vi "test_Get Channel Connection (2010).vi"(8 "error in (no error)":errorcluster) -> (0 "error out":errorcluster)   [LabVIEW 2020, in "Test_Routing Templates.lvlib"]
uses:
  Test_Routing Templates.lvlib
  Connection Lookups/2010 Connection Lookup/2010 Connection Lookup.lvclass
  <vilib>/addons/_JKI Toolkits/Caraya/classes/Assert/Assert Equal Value_Variant.vi
  <vilib>/addons/_JKI Toolkits/Caraya/classes/Assert/Assert Error.vi
  <vilib>/addons/_JKI Toolkits/Caraya/classes/Test/Test.lvclass
  <vilib>/addons/_JKI Toolkits/Caraya/classes/Assert/Assert.lvclass
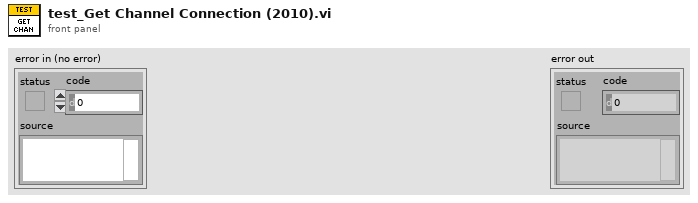
[diagram p1: front panel]
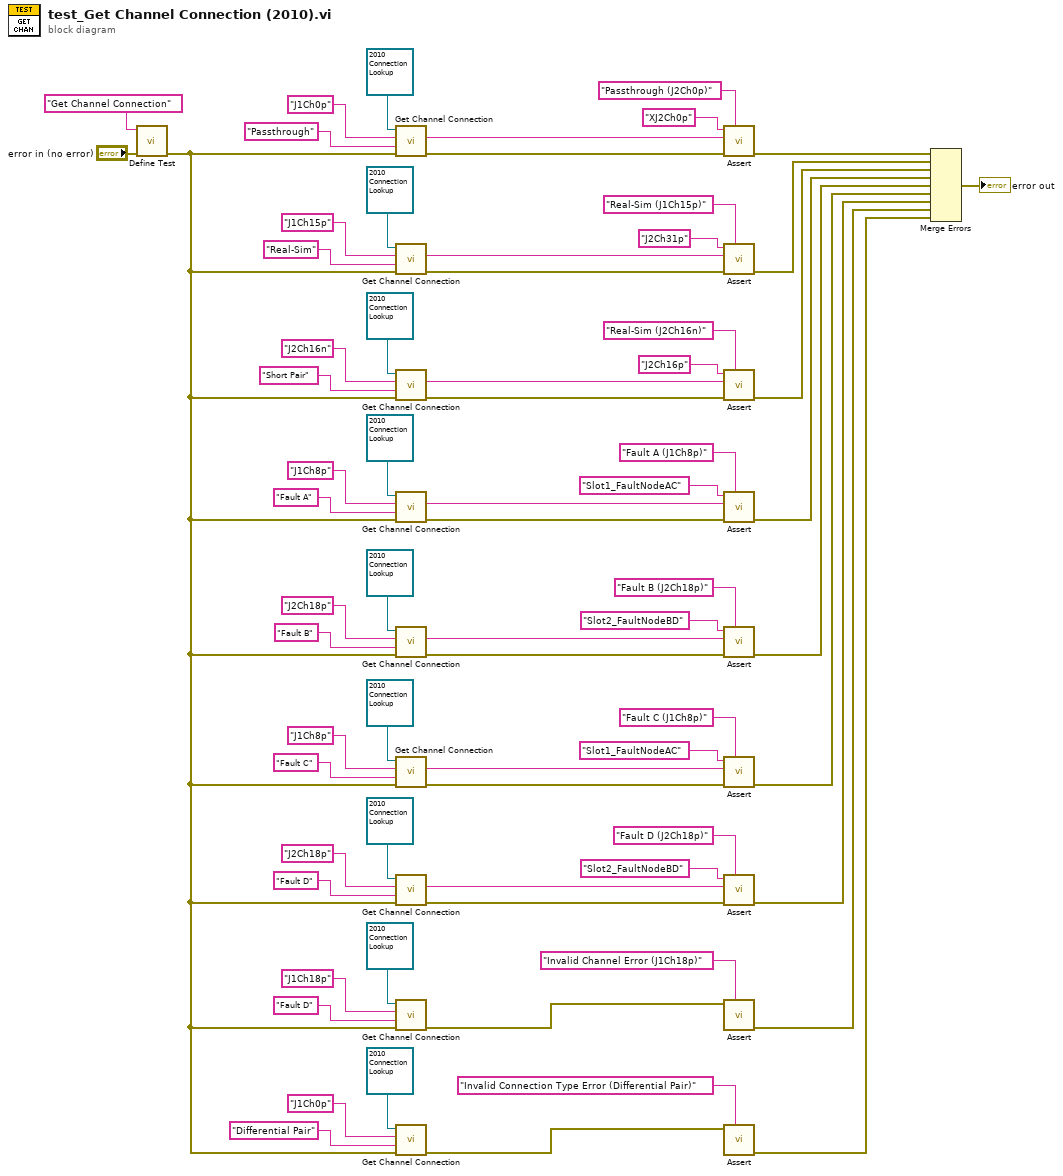
[diagram p0: block diagram]
diagram:
  n1 = call <vilib>:"Define Test.vi"("error in (no error)"="error in (no error)", "Label (VI Title)"="Get Channel Connection") -> ("error out"=w9:errorcluster)  [unwired: 9 in]
  n2 = call-dynamic "Get Channel Connection.vi"("error in (no error)"=w9, "Connection Type"="Passthrough", "Channel"="J1Ch0p", "2010 Connection Lookup in"=refnum<class "2010 Connection Lookup.lvclass"> refnum) -> ("error out"=w70:errorcluster, "Connected Channel"=w63:string)  [unwired: 5 in, 1 out]
  n3 = call-dynamic "Get Channel Connection.vi"("error in (no error)"=w9, "Connection Type"="Real-Sim", "Channel"="J1Ch15p", "2010 Connection Lookup in"=refnum<class "2010 Connection Lookup.lvclass"> refnum) -> ("error out"=w56:errorcluster, "Connected Channel"=w60:string)  [unwired: 5 in, 1 out]
  n4 = call-dynamic "Get Channel Connection.vi"("error in (no error)"=w9, "Connection Type"="Short Pair", "Channel"="J2Ch16n", "2010 Connection Lookup in"=refnum<class "2010 Connection Lookup.lvclass"> refnum) -> ("error out"=w53:errorcluster, "Connected Channel"=w49:string)  [unwired: 5 in, 1 out]
  n5 = call-dynamic "Get Channel Connection.vi"("error in (no error)"=w9, "Connection Type"="Fault A", "Channel"="J1Ch8p", "2010 Connection Lookup in"=refnum<class "2010 Connection Lookup.lvclass"> refnum) -> ("error out"=w42:errorcluster, "Connected Channel"=w46:string)  [unwired: 5 in, 1 out]
  n6 = call-dynamic "Get Channel Connection.vi"("error in (no error)"=w9, "Connection Type"="Fault B", "Channel"="J2Ch18p", "2010 Connection Lookup in"=refnum<class "2010 Connection Lookup.lvclass"> refnum) -> ("error out"=w39:errorcluster, "Connected Channel"=w35:string)  [unwired: 5 in, 1 out]
  n7 = call-dynamic "Get Channel Connection.vi"("error in (no error)"=w9, "Connection Type"="Fault C", "Channel"="J1Ch8p", "2010 Connection Lookup in"=refnum<class "2010 Connection Lookup.lvclass"> refnum) -> ("error out"=w32:errorcluster, "Connected Channel"=w28:string)  [unwired: 5 in, 1 out]
  n8 = call-dynamic "Get Channel Connection.vi"("error in (no error)"=w9, "Connection Type"="Fault D", "Channel"="J2Ch18p", "2010 Connection Lookup in"=refnum<class "2010 Connection Lookup.lvclass"> refnum) -> ("error out"=w21:errorcluster, "Connected Channel"=w25:string)  [unwired: 5 in, 1 out]
  n9 = call-dynamic "Get Channel Connection.vi"("error in (no error)"=w9, "Connection Type"="Fault D", "Channel"="J1Ch18p", "2010 Connection Lookup in"=refnum<class "2010 Connection Lookup.lvclass"> refnum) -> ("error out"=w15:errorcluster)  [unwired: 5 in, 2 out]
  n10 = call-dynamic "Get Channel Connection.vi"("error in (no error)"=w9, "Connection Type"="Differential Pair", "Channel"="J1Ch0p", "2010 Connection Lookup in"=refnum<class "2010 Connection Lookup.lvclass"> refnum) -> ("error out"=w14:errorcluster)  [unwired: 5 in, 2 out]
  n11 = call-poly <vilib>:"Assert.vi"("Label"="Passthrough (J2Ch0p)", "error in (no error)"=w70, "Y"=w63, "X"="XJ2Ch0p" ("Channel")) -> ("error out"=w66:errorcluster)  [unwired: 7 in]
  n12 = call-poly <vilib>:"Assert.vi"("Label"="Real-Sim (J1Ch15p)", "error in (no error)"=w56, "Y"=w60, "X"="J2Ch31p" ("Channel")) -> ("error out"=w8:errorcluster)  [unwired: 7 in]
  n13 = call-poly <vilib>:"Assert.vi"("Label"="Real-Sim (J2Ch16n)", "error in (no error)"=w53, "Y"=w49, "X"="J2Ch16p" ("Channel")) -> ("error out"=w7:errorcluster)  [unwired: 7 in]
  n14 = call-poly <vilib>:"Assert.vi"("Label"="Fault A (J1Ch8p)", "error in (no error)"=w42, "Y"=w46, "X"="Slot1_FaultNodeAC" ("Channel")) -> ("error out"=w6:errorcluster)  [unwired: 7 in]
  n15 = call-poly <vilib>:"Assert.vi"("Label"="Fault B (J2Ch18p)", "error in (no error)"=w39, "Y"=w35, "X"="Slot2_FaultNodeBD" ("Channel")) -> ("error out"=w5:errorcluster)  [unwired: 7 in]
  n16 = call-poly <vilib>:"Assert.vi"("Label"="Fault C (J1Ch8p)", "error in (no error)"=w32, "Y"=w28, "X"="Slot1_FaultNodeAC" ("Channel")) -> ("error out"=w4:errorcluster)  [unwired: 7 in]
  n17 = call-poly <vilib>:"Assert.vi"("Label"="Fault D (J2Ch18p)", "error in (no error)"=w21, "Y"=w25, "X"="Slot2_FaultNodeBD" ("Channel")) -> ("error out"=w3:errorcluster)  [unwired: 7 in]
  n18 = call-poly <vilib>:"Assert.vi"("Label"="Invalid Channel Error (J1Ch18p)", "Error?"=w15) -> ("error out"=w2:errorcluster)  [unwired: 9 in]
  n19 = call-poly <vilib>:"Assert.vi"("Label"="Invalid Connection Type Error (Differential Pair)", "Error?"=w14) -> ("error out"=w1:errorcluster)  [unwired: 9 in]
  n20 = Merge Errors(w66, w8, w7, w6, w5, w4, w3, w2, w1) -> (→"error out":errorcluster)
